vi "PH_PP_CurrentMeas_Start.vi"(0 "connection ID in":refnum<k5>, 2 "NI6071E DAQ Server":string="dveert01.gsi.de", 3 "Port":u16, 5 "error in (no error)":errorcluster) -> (14 "connection ID out":refnum<k5>, 15 "Error unpacking the Data?":bool, 16 "Connection not established":bool, 17 "Received Data Sets":T1[](array[typedef]), 18 "No Task defined?":bool, 19 "error out":errorcluster)   [LabVIEW 2014, in "PH_PP_CurrentMeas.lvlib"]
uses:
  PH_PP_CurrentMeas.lvlib
  PH_PP_CurrentMeas.Command.ctl
  PH_PP_CurrentMeas.CommandCluster.ctl
panel:
  in  "Dummy":T1
  in  "Command":T2=enum."CloseConnection"
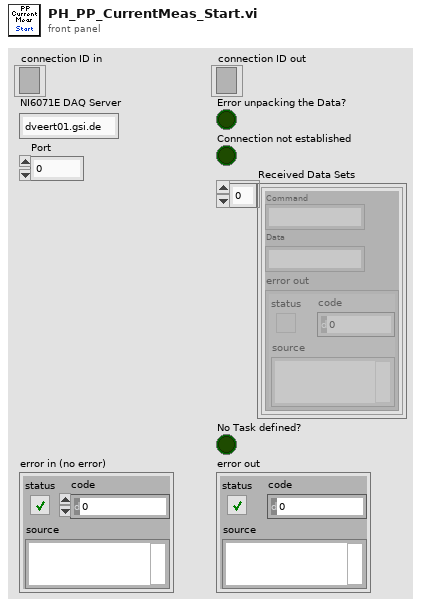
[diagram p1: front panel]
types:
  T1 = typedef "PH_PP_CurrentMeas.lvlib/PH_PP_CurrentMeas.CommandCluster.ctl" = cluster{"Command":string, "Data":string, "error out":errorcluster}
  T2 = typedef "PH_PP_CurrentMeas.lvlib/PH_PP_CurrentMeas.Command.ctl" = enum16{"StartDAQ", "StopDAQ", "GetDAQStatus", "CloseConnection"}
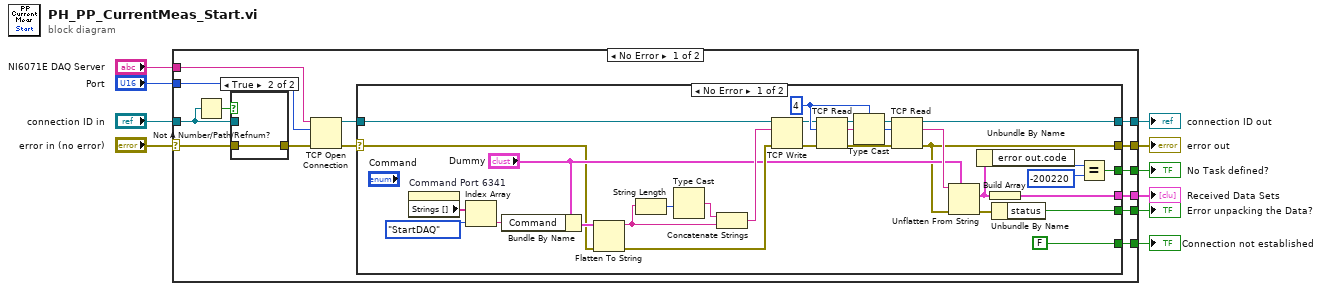
[diagram p0: block diagram]
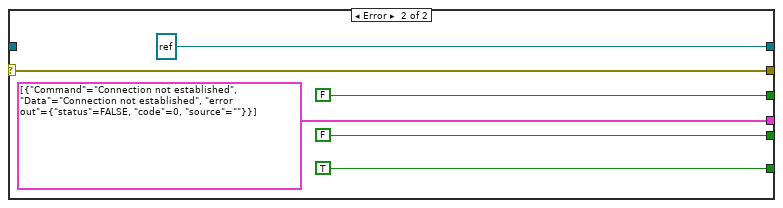
[diagram p2: hidden frame]
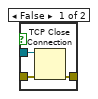
[diagram p3: hidden frame]
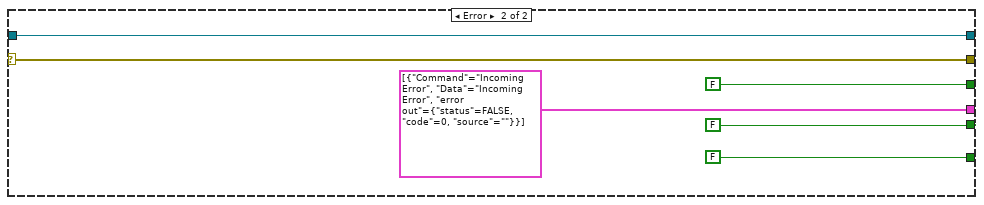
[diagram p4: hidden frame]
diagram:
  n1 = case shown="No Error" "error in (no error)" {
    selector: "error in (no error)" -> [w14 w69]
    tunnel: "connection ID in" -> [w23 w70]
    tunnel: "NI6071E DAQ Server" -> [w20 _]
    tunnel: [w19 w70] -> w8
    tunnel: "Port" -> [w18 _]
    tunnel: [w17 T1[] [{"Command"="Incoming Error", "Data"="Incoming Error", "error out"={"status"=FALSE, "code"=0, "source"=""}}]] -> w6
    tunnel: [w16 FALSE ("status")] -> w5
    tunnel: [w15 w69] -> w4
    tunnel: [w13 FALSE] -> w2
    tunnel: [w11 FALSE ("status")] -> w1
    frame No Error {
      n2 = Not A Number/Path/Refnum?(number/path/refnum=w23) -> (NaN/Path/Refnum?=w24:bool)
      n3 = case shown="True" w24 {
        tunnel: w23 -> [w63 _]
        tunnel: w14 -> [w62 w64]
        tunnel: [w61 w64] -> w22
        frame False {
          n4 = TCP Close Connection(connection ID=w63, error in (no error)=w62) -> (error out=w61:errorcluster)  [unwired: 1 in, 1 out]
        }
        frame True {
        }
      }
      n5 = TCP Open Connection(address=w20, remote port or service name=w18, error in (no error)=w22) -> (connection ID=w21:refnum<k5>, error out=w12:errorcluster)  [unwired: 2 in]
      n6 = case shown="No Error" w12 {
        selector: w12 -> [w30 w60]
        tunnel: w21 -> [w37 _]
        tunnel: [w36 refnum<k5> refnum ("connection ID")] -> w19
        tunnel: [w34 T1[] [{"Command"="Connection not established", "Data"="Connection not established", "error out"={"status"=FALSE, "code"=0, "source"=""}}]] -> w17
        tunnel: [w32 FALSE ("status")] -> w16
        tunnel: [w31 w60] -> w15
        tunnel: [w26 FALSE] -> w13
        tunnel: [FALSE TRUE] -> w11
        frame No Error {
          w43 = 4 ("bytes to read")
          n7 = property on="Command Port 6341" class="Enum (strict)"() -> ("Strings []"=w54:string[])  [unwired: 2 in, 2 out]
          n8 = Index Array(array=w54, index=PH_PP_CurrentMeas.Command."StartDAQ" ("Command")) -> (element=w53:string)
          n9 = Bundle By Name(cluster="Dummy", "Command"=w53) -> (w48:T1)
          n10 = Flatten To String(anything=w48, error in (no error)=w30) -> (data string=w50:string, error out=w47:errorcluster)  [unwired: 2 in, 1 out]
          n11 = String Length(string=w50) -> (length=w51:i32)
          n12 = Type Cast(x=w51) -> (*(type *) &x=w52:string)  [unwired: 1 in]
          n13 = Concatenate Strings(w52, w50) -> (w49:string)
          n14 = TCP Write(connection ID=w37, data in=w49, error in (no error)=w47) -> (connection ID out=w39:refnum<k5>, error out=w40:errorcluster)  [unwired: 1 in, 1 out]
          n15 = TCP Read(connection ID=w39, bytes to read=w43, error in (no error)=w40) -> (connection ID out=w44:refnum<k5>, data out=w41:string, error out=w45:errorcluster)  [unwired: 2 in]
          n16 = Type Cast(type=w43, x=w41) -> (*(type *) &x=w42:i32)
          n17 = TCP Read(connection ID=w44, bytes to read=w42, error in (no error)=w45) -> (connection ID out=w36:refnum<k5>, data out=w46:string, error out=w31:errorcluster)  [unwired: 2 in]
          n18 = Unflatten From String(type="Dummy", binary string=w46, error in (no error)=w31) -> (value=w29:T1, error out=w33:errorcluster)  [unwired: 2 in, 1 out]
          n19 = Unbundle By Name(w29) -> ("error out.code"=w28:i32)
          n20 = Build Array(w29) -> (w34:T1[])
          n21 = Unbundle By Name(w33) -> ("status"=w32:bool)
          n22 = Equal?(x=w28, y=-200220) -> (x = y?=w26:bool)
        }
        frame Error {
        }
      }
    }
    frame Error {
    }
  }
  "connection ID out" <- w8
  "error out" <- w4
  "Received Data Sets" <- w6
  "Error unpacking the Data?" <- w5
  "No Task defined?" <- w2
  "Connection not established" <- w1
